vi "Get flattened data.vi"(8 "error in (no error)":errorcluster, 11 "Double D Element in":refnum<class "Double D Element.lvclass">) -> (0 "error out":errorcluster, 2 "Flattened data":u8[](array[numeric]), 3 "Double D Element out":refnum<class "Double D Element.lvclass">)   [LabVIEW 2018, in "D Datagrid Library.lvlib" / "Double D Element.lvclass"]
uses:
  Double D Element.lvclass
  Double D Element.lvclass/Double D Element.ctl
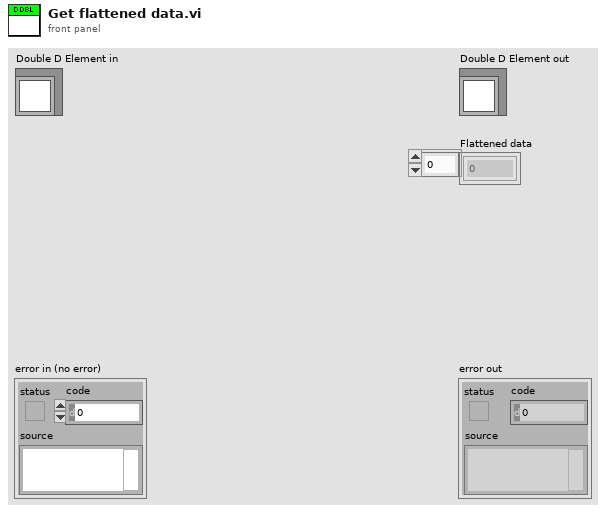
[diagram p1: front panel]
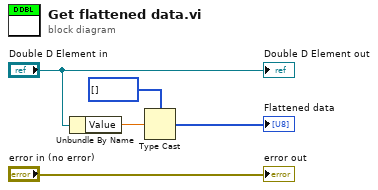
[diagram p0: block diagram]
diagram:
  n1 = Unbundle By Name("Double D Element in") -> ("Value"=w3:dbl)
  n2 = Type Cast(type=u8[] [] ("Flattened data"), x=w3) -> (*(type *) &x=→"Flattened data":u8[])
  "error out" <- "error in (no error)"
  "Double D Element out" <- "Double D Element in"
